vi "CRYSave All.vi"   [LabVIEW 2013]
uses:
  Global/CRYCurve Library Global.vi
panel:
  # "Save All Data(Curves, Values,Results, Waveforms)"
types:
  T1 = cluster{"pattern label":string, "pattern":string}
  T2 = cluster{"pattern label":string, "pattern":string}[]
  T3 = enum16{"Left Button", "Center Button", "Right Button", "Window Close"}
  T4 = typedef "CRYData Cluster.ctl" = cluster{"Name":string, "Curve":cluster{"x":dbl, "y":dbl, "z":dbl}[], "X data":u16, "Y data":u16, "Z data":u16, "X axis":u16, "Y axis":u16, "Z axis":u16, "X unit":string, "Y unit":string, "Z unit":string, "X dB ref":dbl, "Y dB ref":dbl, "Z dB ref":dbl, "single val":bool, "protected":bool, "display X":bool, "display Y":bool, "display Z":bool, "Test Info":string, "Step No.":i32, "Plot Settings":cluster{"Color":u32, "Interpolation":u8, "Point Style":u8, "Line Style":u8, "Point Color":u32, "Line Width":u8, "Bar Plot Style":u8, "Fill To":i16}, "AutoProtect":bool}
  T5 = typedef "CRYWaveform Cluster.ctl" = cluster{"Waveform":cluster{"X0":dbl, "dX":dbl, "Y":sgl[]}, "X data":u16, "Y data":u16, "Y axis":u16, "X unit":string, "Y unit":string, "Y dB ref":dbl, "display Y":bool, "display X":bool, "Overload?":bool, "Test Info":string, "Step No.":i32, "Name":string, "protected":bool, "Sqc history":string[], "Signal Channel ID":i32, "Plot Settings":cluster{"Color":u32, "Interpolation":u8, "Point Style":u8, "Line Style":u8, "Point Color":u32, "Line Width":u8, "Bar Plot Style":u8, "Fill To":i16}, "AutoProtect":bool}
  T6 = typedef "CRYResult Cluster.ctl" = cluster{"Name":string, "Margin":dbl, "unit":string, "Verdict":bool, "Limit":string, "Max/Min":string, "protected":bool, "Step No.":i32, "Test Info":string, "AutoProtect":bool}
  T7 = cluster{"layout":enum16{"rows", "columns"}, "notation":enum16{"sci", "float"}, "precision":i32, "header":enum16{"none", "standard", "custom"}, "custom header":string, "serial no.":bool, "delimiter":enum16{"tab", "comma", "space", "other"}, "other delim":string, "axes":cluster{"x":bool, "y":bool, "z":bool}, "Lot No.":bool, "Operator":bool, "Time Stamp":bool}
  T8 = enum16{"OK", "Yes", "YesNo", "YesNoCancel", "ReplaceAppend"}
  T9 = cluster{"Header format":u16, "Custom Header":string, "Layout":u16, "Delimiter":i32, "Character":string, "notation":u16, "Decimal places":i32, "Comment":string, "axes":cluster{"x":bool, "y":bool, "z":bool}}
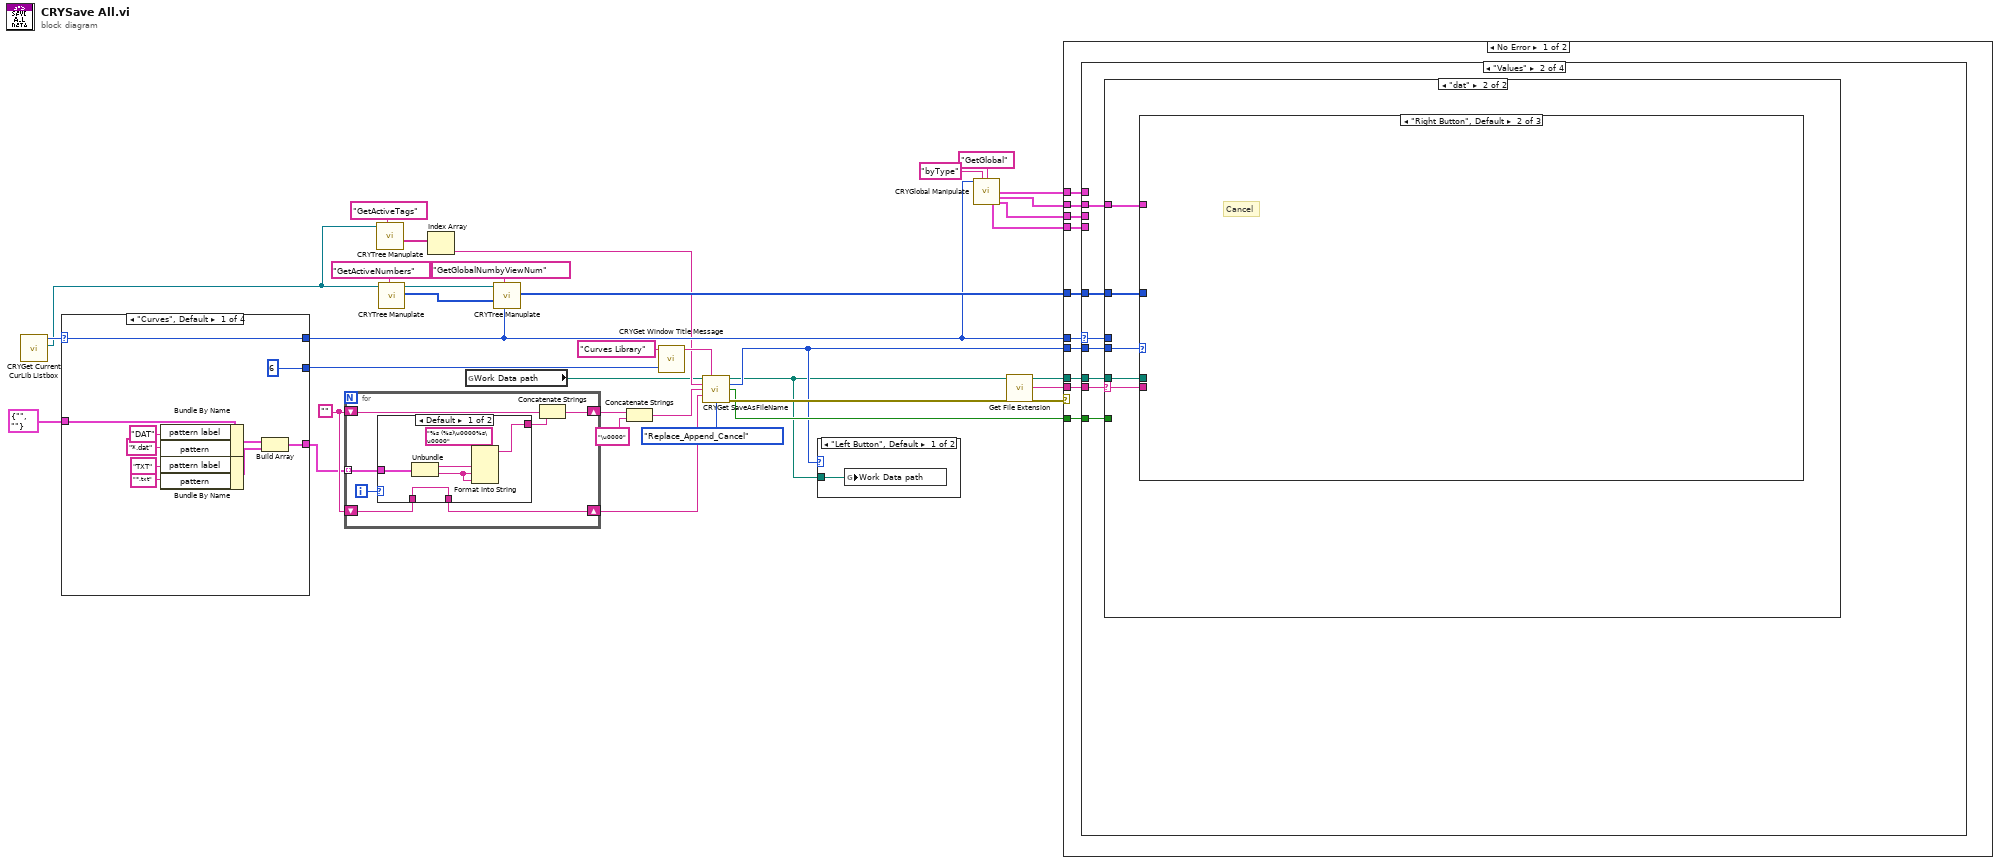
[diagram p0: block diagram]
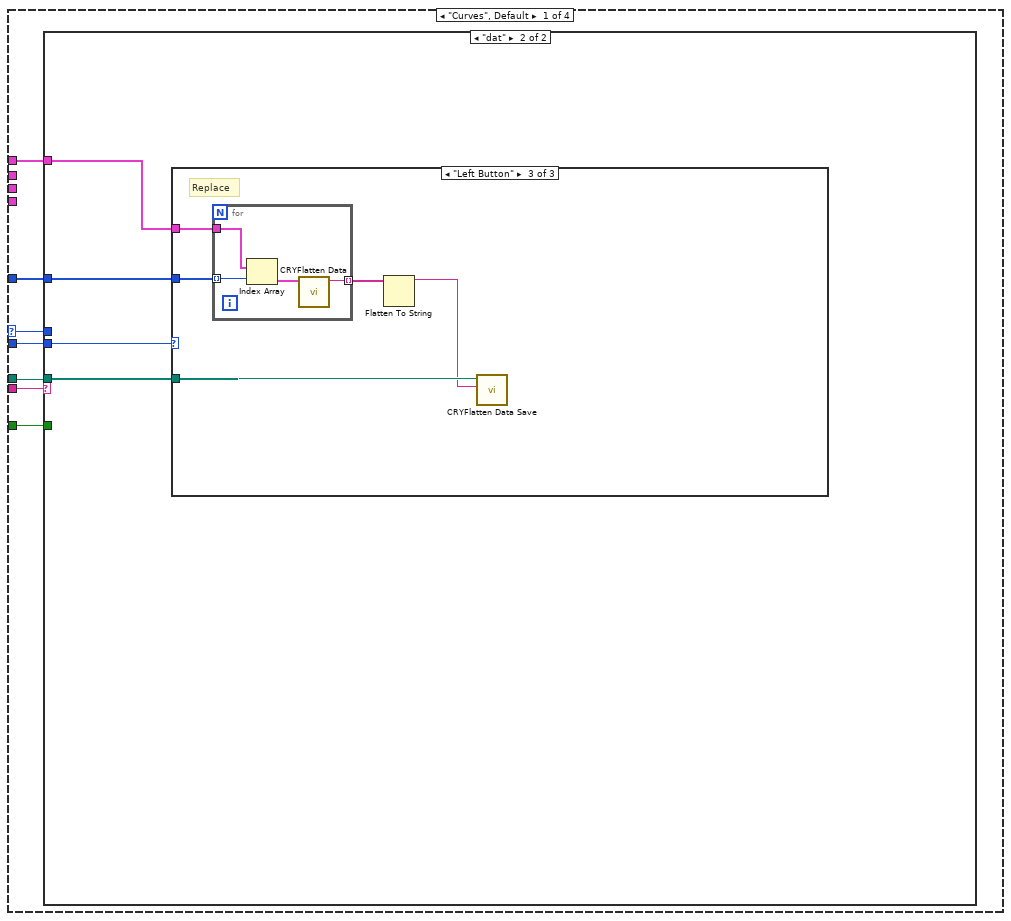
[diagram p3: hidden frame]
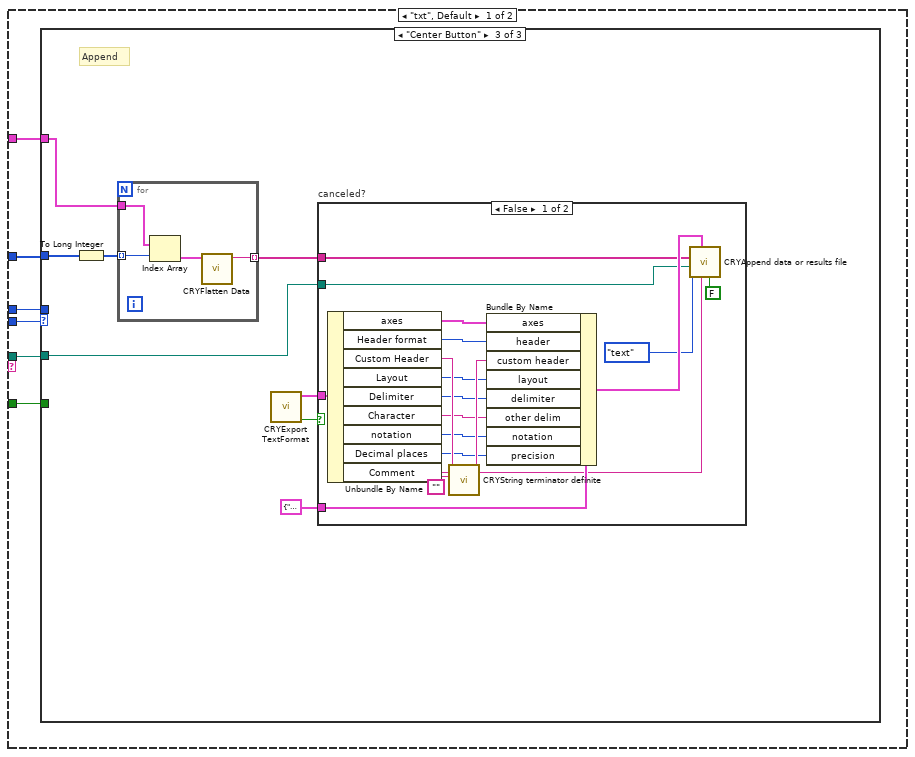
[diagram p4: hidden frame]
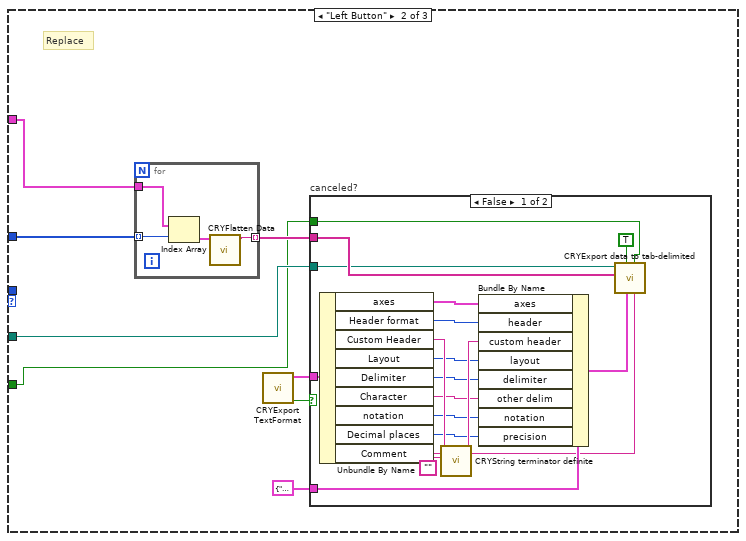
[diagram p6: hidden frame]
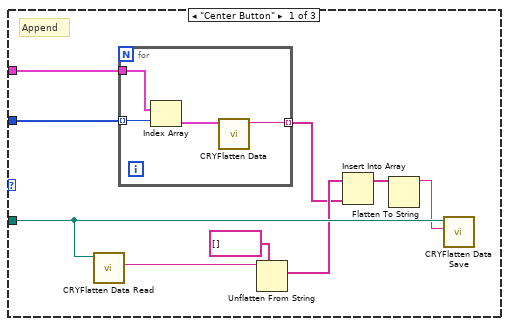
[diagram p9: hidden frame]
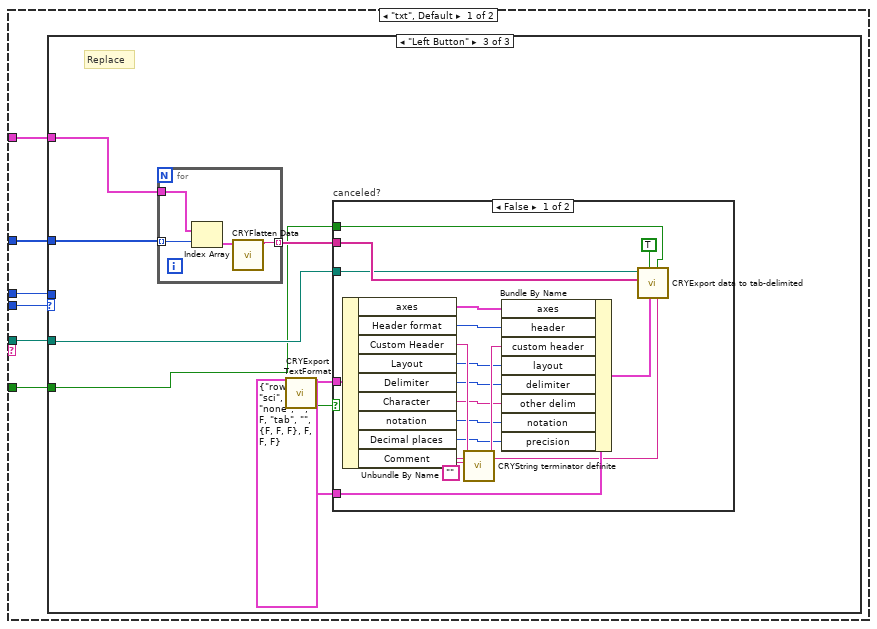
[diagram p11: hidden frame]
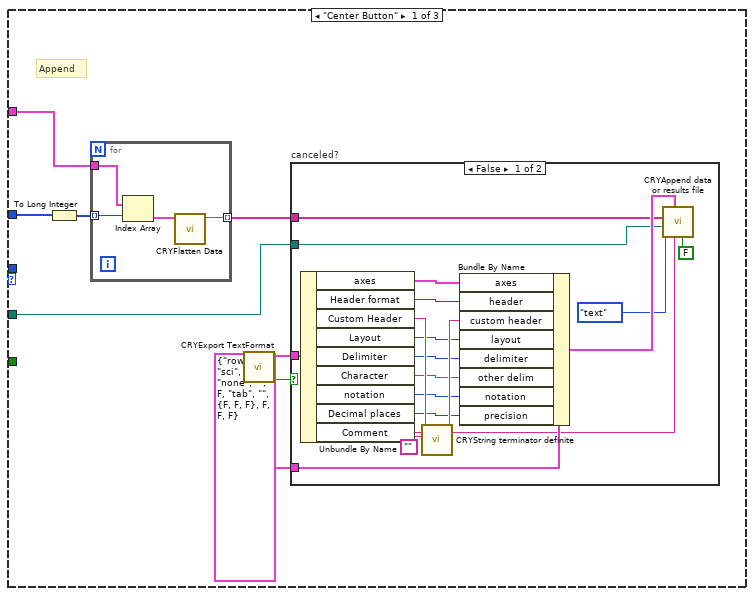
[diagram p12: hidden frame]
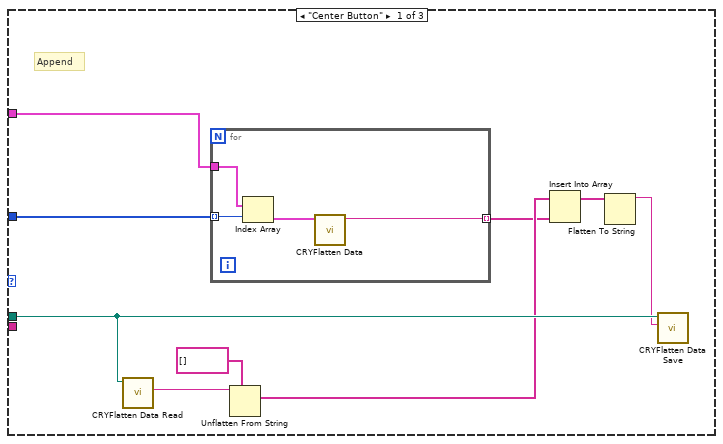
[diagram p16: hidden frame]
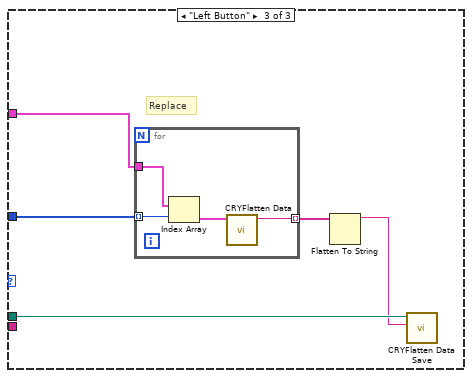
[diagram p17: hidden frame]
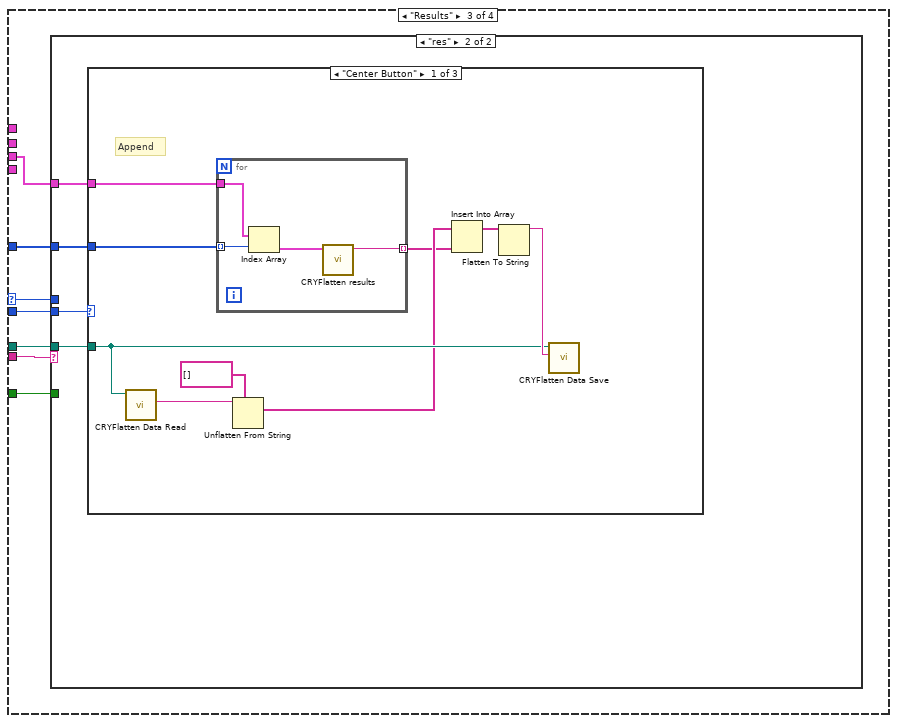
[diagram p18: hidden frame]
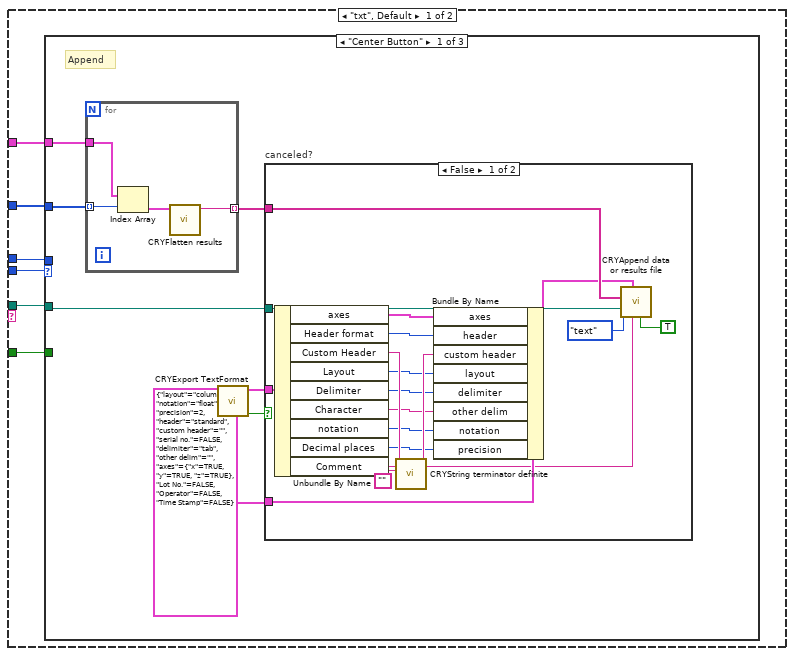
[diagram p19: hidden frame]
diagram:
  w26 = ""
  n1 = call "CRYGet Current CurLib Listbox.vi"() -> ("CurLib Tree"=w6:refnum<vi>, "Type"=w32:enum16{"Curves", "Values", "Results", "WFM"})  [unwired: 9 in, 1 out]
  n2 = case shown="\"Curves\", Default" w32 {
    selector: w32 -> [w46 w56 w66 w76]
    tunnel: [w46 w56 w66 w76] -> w8
    tunnel: [6 ("Error No") 7 ("Error No") 8 ("Error No") 9 ("Error No")] -> w29
    tunnel: T1 {"pattern label"="", "pattern"=""} ("File Types") -> [w37 w47 w58 w68]
    tunnel: [w38 w48 w57 w67] -> w22
    frame "Curves", Default {
      n3 = Bundle By Name(cluster=w37, "pattern label"="DAT" ("pattern (all files)"), "pattern"="*.dat" ("pattern (all files)")) -> (w41:T1)
      n4 = Bundle By Name(cluster=w37, "pattern label"="TXT" ("pattern (all files)"), "pattern"="*.txt" ("pattern (all files)")) -> (w42:T1)
      n5 = Build Array(w41, w42) -> (w38:T2)
    }
    frame "Values" {
      n6 = Bundle By Name(cluster=w47, "pattern label"="DAT" ("pattern (all files)"), "pattern"="*.dat" ("pattern (all files)")) -> (w51:T1)
      n7 = Bundle By Name(cluster=w47, "pattern label"="TXT" ("pattern (all files)"), "pattern"="*.txt" ("pattern (all files)")) -> (w52:T1)
      n8 = Build Array(w51, w52) -> (w48:T2)
    }
    frame "Results" {
      n9 = Bundle By Name(cluster=w58, "pattern label"="RES" ("pattern (all files)"), "pattern"="*.res" ("pattern (all files)")) -> (w61:T1)
      n10 = Bundle By Name(cluster=w58, "pattern label"="TXT" ("pattern (all files)"), "pattern"="*.txt" ("pattern (all files)")) -> (w62:T1)
      n11 = Build Array(w61, w62) -> (w57:T2)
    }
    frame "WFM" {
      n12 = Bundle By Name(cluster=w68, "pattern label"="WAV" ("pattern (all files)"), "pattern"="*.wav" ("pattern (all files)")) -> (w71:T1)
      n13 = Bundle By Name(cluster=w68, "pattern label"="WFM" ("pattern (all files)"), "pattern"="*.wfm" ("pattern (all files)")) -> (w72:T1)
      n14 = Build Array(w71, w72) -> (w67:T2)
    }
  }
  n15 = for {
    tunnel: w22 -> [w83] mode=indexing
    shift-right: [w82] -> w28
    shift-left: w26 -> [w81]
    shift-right: [w78] -> w24
    shift-left: w26 -> [w77]
    i -> [w80]
    n16 = case shown="Default" w80 {
      tunnel: w83 -> [w89 w94]
      tunnel: [w85 w91] -> w79
      tunnel: [w84 w90] -> w78
      tunnel: w77 -> [w84 _]
      frame Default {
        n17 = Unbundle(w89) -> ("pattern label"=w88:string, "pattern"=w86:string)
        n18 = Format Into String(format string="%s (%s)\u0000%s\u0000", w88, w86, w86) -> (resulting string=w85:string)  [unwired: 2 in, 1 out]
      }
      frame 0 {
        n19 = Unbundle(w94) -> ("pattern label"=w90:string, "pattern"=w92:string)
        n20 = Format Into String(format string="%s)\u0000%s\u0000", w92, w92) -> (resulting string=w91:string)  [unwired: 2 in, 1 out]
      }
    }
    n21 = Concatenate Strings(w81, w79) -> (w82:string)
  }
  n22 = call "CRYTree Manuplate.vi"("sAction"="GetActiveTags", "Tree in"=w6) -> ("sData Out"=w5:string[])  [unwired: 6 in, 3 out]
  n23 = call "CRYTree Manuplate.vi"("sAction"="GetActiveNumbers", "Tree in"=w6) -> ("nData Out"=w10:i32[], "Tree Out"=w12:refnum<vi>)  [unwired: 6 in, 2 out]
  n24 = Index Array(array=w5) -> (element=w4:string)  [unwired: 1 in]
  n25 = global read "CRYCurve Library Global.vi" "Work Data path"() -> (w3:path)
  n26 = call "CRYTree Manuplate.vi"("Type"=w8, "sAction"="GetGlobalNumbyViewNum", "nData"=w10, "Tree in"=w12) -> ("nData Out"=w9:i32[])  [unwired: 4 in, 3 out]
  n27 = Concatenate Strings(w28, "\u0000" ("format string")) -> (w25:string)
  n28 = call "CRYGet Window Title Message.vi"("No"=w29, "Kind"="Curves Library") -> ("Multibyte String"=w30:string)  [unwired: 4 in, 5 out]
  n29 = call "CRYGet SaveAsFileName.vi"("Start path"=w3, "TitleName"=w30, "default name"=w4, "pattern (all files)"=w25, "pattern label"=w24, "Enum"=enum16{"Yes_No_Cancel", "Replace_Append_Cancel"}."Replace_Append_Cancel") -> ("Path"=w1:path, "Which Button?"=w2:T3, "Is Replace?"=w21:bool, "error out"=w35:errorcluster)  [unwired: 3 in, 3 out]
  n30 = case shown="\"Left Button\", Default" w2 {
    tunnel: w1 -> [w95 _]
    frame "Left Button", Default {
      n31 = global write "CRYCurve Library Global.vi" "Work Data path"(w95) -> ()
    }
    frame "Right Button" {
    }
  }
  n32 = call "CRYGlobal Manipulate.vi"("Type"=w8, "sOption"="byType", "sAction"="GetGlobal") -> ("Curves Out"=w16:T4[], "Values Out"=w15:T4[], "WFM Out"=w13:T5[], "Results Out"=w14:T6[])  [unwired: 6 in, 3 out]
  n33 = call <vilib>:"Get File Extension.vi"("error in (no error)"=w35, "file"=w1) -> ("error out"=w20:errorcluster, "lowercase file extension"=w33:string, "dup file"=w34:path)  [unwired: 7 out]
  n34 = case shown="No Error" w20 {
    tunnel: w2 -> [w105 _]
    tunnel: w8 -> [w104 _]
    tunnel: w34 -> [w103 _]
    tunnel: w33 -> [w102 _]
    tunnel: w9 -> [w101 _]
    tunnel: w21 -> [w100 _]
    tunnel: w16 -> [w99 _]
    tunnel: w15 -> [w98 _]
    tunnel: w14 -> [w97 _]
    tunnel: w13 -> [w96 _]
    frame No Error {
      n35 = case shown="\"Values\"" w104 {
        selector: w104 -> [w108 w207 w307 _]
        tunnel: w105 -> [w112 w211 w310 w406]
        tunnel: w101 -> [w111 w210 w311 w407]
        tunnel: w103 -> [w110 w209 w309 w405]
        tunnel: w102 -> [w109 w208 w308 w404]
        tunnel: w100 -> [w107 w206 w306 _]
        tunnel: w99 -> [w106 _ _ _]
        tunnel: w98 -> [_ w205 _ _]
        tunnel: w97 -> [_ _ w305 _]
        tunnel: w96 -> [_ _ _ w403]
        frame "Curves", Default {
          n36 = case shown="\"dat\"" w109 {
            tunnel: w112 -> [w117 w182]
            tunnel: w111 -> [w118 w181]
            tunnel: w110 -> [w116 w180]
            tunnel: w108 -> [w115 _]
            tunnel: w107 -> [w114 _]
            tunnel: w106 -> [w113 w179]
            frame "txt", Default {
              n37 = case shown="\"Center Button\"" w117 {
                tunnel: w118 -> [_ w126 w155]
                tunnel: w116 -> [_ w123 w150]
                tunnel: w115 -> [_ _ _]
                tunnel: w114 -> [_ w120 _]
                tunnel: w113 -> [_ w119 w149]
                frame "Right Button", Default {
                  # "Cancel"
                }
                frame "Left Button" {
                  # "Replace"
                  n38 = for {
                    tunnel: w126 -> [w148] mode=indexing
                    tunnel: w119 -> [w147]
                    tunnel: [w145] -> w121 mode=indexing
                    n39 = Index Array(array=w147, index=w148) -> (element=w146:T4)
                    n40 = call "CRYFlatten Data.vi"("Datum"=w146) -> ("Data flattened"=w145:string)  [unwired: 10 in]
                  }
                  n41 = call "CRYExport TextFormat.vi"() -> ("Canceled"=w125:bool, "Export format"=w124:T9)  [unwired: 10 in]
                  n42 = case "canceled?" shown="False" w125 {
                    tunnel: w124 -> [w144 _]
                    tunnel: T7 {"layout"=enum."rows", "notation"=enum."sci", "precision"=0, "header"=enum."none", "custom header"="", "serial no."=FALSE, "delimiter"=enum."tab", "other delim"="", "axes"={"x"=FALSE, "y"=FALSE, "z"=FALSE}, "Lot No."=FALSE, "Operator"=FALSE, "Time Stamp"=FALSE} ("input cluster") -> [w135 _]
                    tunnel: w123 -> [w129 _]
                    tunnel: w121 -> [w130 _]
                    tunnel: w120 -> [w127 _]
                    frame False {
                      n43 = Unbundle By Name(w144) -> ("axes"=w131:cluster{"x":bool, "y":bool, "z":bool}, "Header format"=w136:u16, "Custom Header"=w143:string, "Layout"=w137:u16, "Delimiter"=w138:i32, "Character"=w139:string, "notation"=w140:u16, "Decimal places"=w141:i32, "Comment"=w132:string)
                      n44 = call "CRYString terminator definite.vi"("Terminator"="", "String in"=w143) -> ("String out"=w142:string)  [unwired: 9 in]
                      n45 = Bundle By Name(cluster=w135, "axes"=w131, "header"=w136, "custom header"=w142, "layout"=w137, "delimiter"=w138, "other delim"=w139, "notation"=w140, "precision"=w141) -> (w134:T7)
                      n46 = call "CRYExport data to tab-delimited.vi"("Comment"=w132, "File exists & overwrite (F)"=w127, "Format info"=w134, "Use format info? (F)"=TRUE, "data series"=w130, "File path (not wired: dialogue)"=w129) -> ()  [unwired: 3 in, 3 out]
                    }
                    frame True {
                    }
                  }
                }
                frame "Center Button" {
                  # "Append"
                  n47 = To Long Integer(number=w155) -> (32bit integer=w156:i32[])
                  n48 = for {
                    tunnel: w156 -> [w178] mode=indexing
                    tunnel: w149 -> [w177]
                    tunnel: [w176] -> w151 mode=indexing
                    n49 = Index Array(array=w177, index=w178) -> (element=w175:T4)
                    n50 = call "CRYFlatten Data.vi"("Datum"=w175) -> ("Data flattened"=w176:string)  [unwired: 10 in]
                  }
                  n51 = call "CRYExport TextFormat.vi"() -> ("Canceled"=w154:bool, "Export format"=w153:T9)  [unwired: 10 in]
                  n52 = case "canceled?" shown="False" w154 {
                    tunnel: w153 -> [w174 _]
                    tunnel: T7 {"layout"=enum."rows", "notation"=enum."sci", "precision"=0, "header"=enum."none", "custom header"="", "serial no."=FALSE, "delimiter"=enum."tab", "other delim"="", "axes"={"x"=FALSE, "y"=FALSE, "z"=FALSE}, "Lot No."=FALSE, "Operator"=FALSE, "Time Stamp"=FALSE} ("input cluster") -> [w165 _]
                    tunnel: w150 -> [w157 _]
                    tunnel: w151 -> [w160 _]
                    frame False {
                      n53 = Unbundle By Name(w174) -> ("axes"=w161:cluster{"x":bool, "y":bool, "z":bool}, "Header format"=w166:u16, "Custom Header"=w173:string, "Layout"=w167:u16, "Delimiter"=w168:i32, "Character"=w169:string, "notation"=w170:u16, "Decimal places"=w171:i32, "Comment"=w162:string)
                      n54 = call "CRYString terminator definite.vi"("Terminator"="", "String in"=w173) -> ("String out"=w172:string)  [unwired: 9 in]
                      n55 = Bundle By Name(cluster=w165, "axes"=w161, "header"=w166, "custom header"=w172, "layout"=w167, "delimiter"=w168, "other delim"=w169, "notation"=w170, "precision"=w171) -> (w164:T7)
                      n56 = call "CRYAppend data or results file.vi"("Is results? (F)"=FALSE, "Comment"=w162, "Format info"=w164, "data format"=enum16{"text", "DAT"}."text", "Datafile path"=w157, "Curves list to save"=w160) -> ()  [unwired: 5 in, 1 out]
                    }
                    frame True {
                    }
                  }
                }
              }
            }
            frame "dat" {
              n57 = case shown="\"Left Button\"" w182 {
                tunnel: w181 -> [w191 _ w200]
                tunnel: w179 -> [w185 _ w198]
                tunnel: w180 -> [w190 _ w197]
                frame "Center Button" {
                  # "Append"
                  n58 = call "CRYFlatten Data Read.vi"("Path In"=w190) -> ("Flatten Data Out"=w189:string)  [unwired: 1 in, 7 out]
                  n59 = for {
                    tunnel: w191 -> [w195] mode=indexing
                    tunnel: w185 -> [w194]
                    tunnel: [w192] -> w184 mode=indexing
                    n60 = Index Array(array=w194, index=w195) -> (element=w193:T4)
                    n61 = call "CRYFlatten Data.vi"("Datum"=w193) -> ("Data flattened"=w192:string)  [unwired: 10 in]
                  }
                  n62 = Unflatten From String(type=string[] [] ("value"), binary string=w189) -> (value=w186:string[])  [unwired: 1 in, 4 out]
                  n63 = Insert Into Array(array=w186, new element=w184) -> (w187:string[])  [unwired: 1 in]
                  n64 = Flatten To String(anything=w187) -> (data string=w188:string)  [unwired: 1 in, 4 out]
                  n65 = call "CRYFlatten Data Save.vi"("Any Flatten Data"=w188, "Path In"=w190) -> ()  [unwired: 1 in, 7 out]
                }
                frame "Right Button", Default {
                  # "Cancel"
                }
                frame "Left Button" {
                  # "Replace"
                  n66 = for {
                    tunnel: w200 -> [w204] mode=indexing
                    tunnel: w198 -> [w203]
                    tunnel: [w201] -> w199 mode=indexing
                    n67 = Index Array(array=w203, index=w204) -> (element=w202:T4)
                    n68 = call "CRYFlatten Data.vi"("Datum"=w202) -> ("Data flattened"=w201:string)  [unwired: 10 in]
                  }
                  n69 = Flatten To String(anything=w199) -> (data string=w196:string)  [unwired: 1 in, 4 out]
                  n70 = call "CRYFlatten Data Save.vi"("Any Flatten Data"=w196, "Path In"=w197) -> ()  [unwired: 1 in, 7 out]
                }
              }
            }
          }
        }
        frame "Values" {
          n71 = case shown="\"dat\"" w208 {
            selector: w208 -> [_ w278]
            tunnel: w211 -> [w217 w282]
            tunnel: w210 -> [w214 w281]
            tunnel: w209 -> [w216 w280]
            tunnel: w207 -> [w215 _]
            tunnel: w206 -> [w213 _]
            tunnel: w205 -> [w212 w279]
            frame "txt", Default {
              n72 = case shown="\"Left Button\"" w217 {
                tunnel: w214 -> [w219 _ w251]
                tunnel: w216 -> [w220 _ w250]
                tunnel: w215 -> [_ _ _]
                tunnel: w213 -> [_ _ w249]
                tunnel: w212 -> [w218 _ w248]
                frame "Center Button" {
                  # "Append"
                  n73 = To Long Integer(number=w219) -> (32bit integer=w225:i32[])
                  n74 = for {
                    tunnel: w225 -> [w247] mode=indexing
                    tunnel: w218 -> [w246]
                    tunnel: [w245] -> w221 mode=indexing
                    n75 = Index Array(array=w246, index=w247) -> (element=w244:T4)
                    n76 = call "CRYFlatten Data.vi"("Datum"=w244) -> ("Data flattened"=w245:string)  [unwired: 10 in]
                  }
                  n77 = call "CRYExport TextFormat.vi"() -> ("Canceled"=w224:bool, "Export format"=w223:T9)  [unwired: 10 in]
                  n78 = case "canceled?" shown="False" w224 {
                    tunnel: w223 -> [w243 _]
                    tunnel: T7 {"layout"=enum."rows", "notation"=enum."sci", "precision"=0, "header"=enum."none", "custom header"="", "serial no."=FALSE, "delimiter"=enum."tab", "other delim"="", "axes"={"x"=FALSE, "y"=FALSE, "z"=FALSE}, "Lot No."=FALSE, "Operator"=FALSE, "Time Stamp"=FALSE} ("input cluster") -> [w234 _]
                    tunnel: w220 -> [w226 _]
                    tunnel: w221 -> [w229 _]
                    frame False {
                      n79 = Unbundle By Name(w243) -> ("axes"=w230:cluster{"x":bool, "y":bool, "z":bool}, "Header format"=w235:u16, "Custom Header"=w242:string, "Layout"=w236:u16, "Delimiter"=w237:i32, "Character"=w238:string, "notation"=w239:u16, "Decimal places"=w240:i32, "Comment"=w231:string)
                      n80 = call "CRYString terminator definite.vi"("Terminator"="", "String in"=w242) -> ("String out"=w241:string)  [unwired: 9 in]
                      n81 = Bundle By Name(cluster=w234, "axes"=w230, "header"=w235, "custom header"=w241, "layout"=w236, "delimiter"=w237, "other delim"=w238, "notation"=w239, "precision"=w240) -> (w233:T7)
                      n82 = call "CRYAppend data or results file.vi"("Is results? (F)"=FALSE, "Comment"=w231, "Format info"=w233, "data format"=enum16{"text", "DAT"}."text", "Datafile path"=w226, "Curves list to save"=w229) -> ()  [unwired: 5 in, 1 out]
                    }
                    frame True {
                    }
                  }
                }
                frame "Right Button", Default {
                  # "Cancel"
                }
                frame "Left Button" {
                  # "Replace"
                  n83 = for {
                    tunnel: w251 -> [w277] mode=indexing
                    tunnel: w248 -> [w276]
                    tunnel: [w274] -> w252 mode=indexing
                    n84 = Index Array(array=w276, index=w277) -> (element=w275:T4)
                    n85 = call "CRYFlatten Data.vi"("Datum"=w275) -> ("Data flattened"=w274:string)  [unwired: 10 in]
                  }
                  n86 = call "CRYExport TextFormat.vi"() -> ("Canceled"=w255:bool, "Export format"=w254:T9)  [unwired: 10 in]
                  n87 = case "canceled?" shown="False" w255 {
                    tunnel: w254 -> [w273 _]
                    tunnel: T7 {"layout"=enum."rows", "notation"=enum."sci", "precision"=0, "header"=enum."none", "custom header"="", "serial no."=FALSE, "delimiter"=enum."tab", "other delim"="", "axes"={"x"=FALSE, "y"=FALSE, "z"=FALSE}, "Lot No."=FALSE, "Operator"=FALSE, "Time Stamp"=FALSE} ("input cluster") -> [w264 _]
                    tunnel: w250 -> [w258 _]
                    tunnel: w252 -> [w259 _]
                    tunnel: w249 -> [w256 _]
                    frame False {
                      n88 = Unbundle By Name(w273) -> ("axes"=w260:cluster{"x":bool, "y":bool, "z":bool}, "Header format"=w265:u16, "Custom Header"=w272:string, "Layout"=w266:u16, "Delimiter"=w267:i32, "Character"=w268:string, "notation"=w269:u16, "Decimal places"=w270:i32, "Comment"=w261:string)
                      n89 = call "CRYString terminator definite.vi"("Terminator"="", "String in"=w272) -> ("String out"=w271:string)  [unwired: 9 in]
                      n90 = Bundle By Name(cluster=w264, "axes"=w260, "header"=w265, "custom header"=w271, "layout"=w266, "delimiter"=w267, "other delim"=w268, "notation"=w269, "precision"=w270) -> (w263:T7)
                      n91 = call "CRYExport data to tab-delimited.vi"("Comment"=w261, "File exists & overwrite (F)"=w256, "Format info"=w263, "Use format info? (F)"=TRUE, "data series"=w259, "File path (not wired: dialogue)"=w258) -> ()  [unwired: 3 in, 3 out]
                    }
                    frame True {
                    }
                  }
                }
              }
            }
            frame "dat" {
              n92 = case shown="\"Right Button\", Default" w282 {
                tunnel: w281 -> [w291 _ w300]
                tunnel: w280 -> [w289 _ w298]
                tunnel: w279 -> [w283 _ w296]
                tunnel: w278 -> [_ _ _]
                frame "Center Button" {
                  # "Append"
                  n93 = call "CRYFlatten Data Read.vi"("Path In"=w289) -> ("Flatten Data Out"=w290:string)  [unwired: 1 in, 7 out]
                  n94 = for {
                    tunnel: w291 -> [w295] mode=indexing
                    tunnel: [w292] -> w284 mode=indexing
                    tunnel: w283 -> [w294]
                    n95 = Index Array(array=w294, index=w295) -> (element=w293:T4)
                    n96 = call "CRYFlatten Data.vi"("Datum"=w293) -> ("Data flattened"=w292:string)  [unwired: 10 in]
                  }
                  n97 = Unflatten From String(type=string[] [] ("value"), binary string=w290) -> (value=w285:string[])  [unwired: 1 in, 4 out]
                  n98 = Insert Into Array(array=w285, new element=w284) -> (w287:string[])  [unwired: 1 in]
                  n99 = Flatten To String(anything=w287) -> (data string=w288:string)  [unwired: 1 in, 4 out]
                  n100 = call "CRYFlatten Data Save.vi"("Any Flatten Data"=w288, "Path In"=w289) -> ()  [unwired: 1 in, 7 out]
                }
                frame "Right Button", Default {
                  # "Cancel"
                }
                frame "Left Button" {
                  # "Replace"
                  n101 = for {
                    tunnel: w300 -> [w304] mode=indexing
                    tunnel: [w301] -> w299 mode=indexing
                    tunnel: w296 -> [w303]
                    n102 = Index Array(array=w303, index=w304) -> (element=w302:T4)
                    n103 = call "CRYFlatten Data.vi"("Datum"=w302) -> ("Data flattened"=w301:string)  [unwired: 10 in]
                  }
                  n104 = Flatten To String(anything=w299) -> (data string=w297:string)  [unwired: 1 in, 4 out]
                  n105 = call "CRYFlatten Data Save.vi"("Any Flatten Data"=w297, "Path In"=w298) -> ()  [unwired: 1 in, 7 out]
                }
              }
            }
          }
        }
        frame "Results" {
          n106 = case shown="\"res\"" w308 {
            tunnel: w305 -> [w317 w380]
            tunnel: w311 -> [w316 w379]
            tunnel: w310 -> [w315 w378]
            tunnel: w309 -> [w313 w377]
            tunnel: w307 -> [w314 _]
            tunnel: w306 -> [w312 _]
            frame "txt", Default {
              n107 = case shown="\"Center Button\"" w315 {
                tunnel: w316 -> [w324 _ w354]
                tunnel: w317 -> [w323 _ w353]
                tunnel: w313 -> [w319 _ w350]
                tunnel: w314 -> [_ _ _]
                tunnel: w312 -> [_ _ w347]
                frame "Center Button" {
                  # "Append"
                  n108 = for {
                    tunnel: w324 -> [w346] mode=indexing
                    tunnel: w323 -> [w345]
                    tunnel: [w343] -> w320 mode=indexing
                    n109 = Index Array(array=w345, index=w346) -> (element=w344:T6)
                    n110 = call "CRYFlatten results.vi"("Result in"=w344) -> ("Flatten Result"=w343:string)  [unwired: 10 in]
                  }
                  n111 = call "CRYExport TextFormat.vi"() -> ("Canceled"=w322:bool, "Export format"=w321:T9)  [unwired: 10 in]
                  n112 = case "canceled?" shown="False" w322 {
                    tunnel: w321 -> [w342 _]
                    tunnel: T7 {"layout"=enum."columns", "notation"=enum."float", "precision"=2, "header"=enum."standard", "custom header"="", "serial no."=FALSE, "delimiter"=enum."tab", "other delim"="", "axes"={"x"=TRUE, "y"=TRUE, "z"=TRUE}, "Lot No."=FALSE, "Operator"=FALSE, "Time Stamp"=FALSE} ("Format info") -> [w333 _]
                    tunnel: w319 -> [w326 _]
                    tunnel: w320 -> [w329 _]
                    frame False {
                      n113 = Unbundle By Name(w342) -> ("axes"=w330:cluster{"x":bool, "y":bool, "z":bool}, "Header format"=w334:u16, "Custom Header"=w341:string, "Layout"=w335:u16, "Delimiter"=w336:i32, "Character"=w337:string, "notation"=w338:u16, "Decimal places"=w339:i32, "Comment"=w331:string)
                      n114 = call "CRYString terminator definite.vi"("Terminator"="", "String in"=w341) -> ("String out"=w340:string)  [unwired: 9 in]
                      n115 = Bundle By Name(cluster=w333, "axes"=w330, "header"=w334, "custom header"=w340, "layout"=w335, "delimiter"=w336, "other delim"=w337, "notation"=w338, "precision"=w339) -> (w325:T7)
                      n116 = call "CRYAppend data or results file.vi"("Is results? (F)"=TRUE, "Comment"=w331, "Format info"=w325, "data format"=enum16{"text", "DAT"}."text", "Datafile path"=w326, "Curves list to save"=w329) -> ()  [unwired: 5 in, 1 out]
                    }
                    frame True {
                    }
                  }
                }
                frame "Right Button", Default {
                  # "Cancel"
                }
                frame "Left Button" {
                  # "Replace"
                  n117 = for {
                    tunnel: w354 -> [w376] mode=indexing
                    tunnel: w353 -> [w375]
                    tunnel: [w373] -> w349 mode=indexing
                    n118 = Index Array(array=w375, index=w376) -> (element=w374:T6)
                    n119 = call "CRYFlatten results.vi"("Result in"=w374) -> ("Flatten Result"=w373:string)  [unwired: 10 in]
                  }
                  n120 = call "CRYExport TextFormat.vi"() -> ("Canceled"=w352:bool, "Export format"=w351:T9)  [unwired: 10 in]
                  n121 = case "canceled?" shown="False" w352 {
                    tunnel: w351 -> [w372 _]
                    tunnel: T7 {"layout"=enum."rows", "notation"=enum."sci", "precision"=0, "header"=enum."none", "custom header"="", "serial no."=FALSE, "delimiter"=enum."tab", "other delim"="", "axes"={"x"=FALSE, "y"=FALSE, "z"=FALSE}, "Lot No."=FALSE, "Operator"=FALSE, "Time Stamp"=FALSE} ("Format info") -> [w363 _]
                    tunnel: w350 -> [w356 _]
                    tunnel: w349 -> [w358 _]
                    tunnel: w347 -> [w355 _]
                    frame False {
                      n122 = Unbundle By Name(w372) -> ("axes"=w360:cluster{"x":bool, "y":bool, "z":bool}, "Header format"=w364:u16, "Custom Header"=w371:string, "Layout"=w365:u16, "Delimiter"=w366:i32, "Character"=w367:string, "notation"=w368:u16, "Decimal places"=w369:i32, "Comment"=w361:string)
                      n123 = call "CRYString terminator definite.vi"("Terminator"="", "String in"=w371) -> ("String out"=w370:string)  [unwired: 9 in]
                      n124 = Bundle By Name(cluster=w363, "axes"=w360, "header"=w364, "custom header"=w370, "layout"=w365, "delimiter"=w366, "other delim"=w367, "notation"=w368, "precision"=w369) -> (w357:T7)
                      n125 = call "CRYResult save as text.vi"("File exists & overwrite (F)"=w355, "Comment"=w361, "File format"=enum16{"text", "RES"}."text", "Format info"=w357, "Path"=w356, "Results stack, flat"=w358) -> ()  [unwired: 6 in]
                    }
                    frame True {
                    }
                  }
                }
              }
            }
            frame "res" {
              n126 = case shown="\"Center Button\"" w378 {
                tunnel: w379 -> [w389 _ w398]
                tunnel: w380 -> [w385 _ w396]
                tunnel: w377 -> [w386 _ w395]
                frame "Center Button" {
                  # "Append"
                  n127 = call "CRYFlatten Data Read.vi"("Path In"=w386) -> ("Flatten Data Out"=w387:string)  [unwired: 1 in, 7 out]
                  n128 = for {
                    tunnel: w389 -> [w393] mode=indexing
                    tunnel: [w391] -> w382 mode=indexing
                    tunnel: w385 -> [w392]
                    n129 = Index Array(array=w392, index=w393) -> (element=w390:T6)
                    n130 = call "CRYFlatten results.vi"("Result in"=w390) -> ("Flatten Result"=w391:string)  [unwired: 10 in]
                  }
                  n131 = Unflatten From String(type=string[] [] ("value"), binary string=w387) -> (value=w383:string[])  [unwired: 1 in, 4 out]
                  n132 = Insert Into Array(array=w383, new element=w382) -> (w384:string[])  [unwired: 1 in]
                  n133 = Flatten To String(anything=w384) -> (data string=w388:string)  [unwired: 1 in, 4 out]
                  n134 = call "CRYFlatten Data Save.vi"("Any Flatten Data"=w388, "Path In"=w386) -> ()  [unwired: 1 in, 7 out]
                }
                frame "Right Button", Default {
                  # "Cancel"
                }
                frame "Left Button" {
                  # "Replace"
                  n135 = for {
                    tunnel: w398 -> [w402] mode=indexing
                    tunnel: [w399] -> w397 mode=indexing
                    tunnel: w396 -> [w401]
                    n136 = Index Array(array=w401, index=w402) -> (element=w400:T6)
                    n137 = call "CRYFlatten results.vi"("Result in"=w400) -> ("Flatten Result"=w399:string)  [unwired: 10 in]
                  }
                  n138 = Flatten To String(anything=w397) -> (data string=w394:string)  [unwired: 1 in, 4 out]
                  n139 = call "CRYFlatten Data Save.vi"("Any Flatten Data"=w394, "Path In"=w395) -> ()  [unwired: 1 in, 7 out]
                }
              }
            }
          }
        }
        frame "WFM" {
          n140 = case shown="\"wav\", Default" w404 {
            tunnel: w403 -> [w411 w460]
            tunnel: w407 -> [w410 w459]
            tunnel: w406 -> [w409 w458]
            tunnel: w405 -> [w408 w457]
            frame "wav", Default {
              n141 = case shown="\"Left Button\"" w409 {
                tunnel: w410 -> [_ _ w418]
                tunnel: w411 -> [_ _ w420]
                tunnel: w408 -> [_ _ w419]
                frame "Center Button" {
                  n142 = call "CRYGet Error Message.vi"("Error No"=5, "Kind"="Curves Library") -> ("Message"=w412:string, "Window Title"=w413:string)  [unwired: 4 in, 4 out]
                  n143 = call "CRYMessage Dialog.vi"("Window Title"=w413, "YesNoCancel"=T8."OK", "Message Content"=w412) -> ()  [unwired: 7 in, 2 out]
                }
                frame "Right Button", Default {
                  # "Cancel"
                }
                frame "Left Button" {
                  # "Replace"
                  n144 = Array Size(array=w418) -> (size(s)=w417:i32)
                  n145 = case shown="1, 2" w417 {
                    selector: w417 -> [w425 _]
                    tunnel: w418 -> [w421 _]
                    tunnel: w420 -> [w426 _]
                    tunnel: w419 -> [w428 _]
                    frame 1, 2 {
                      n146 = case shown="1, Default" w425 {
                        tunnel: [w437 w450] -> w429
                        tunnel: w426 -> [w436 w449]
                        tunnel: [w435 w446] -> w424
                        tunnel: [u32 1 ("Channel") u32 2 ("Channel")] -> w422
                        tunnel: w421 -> [w433 w444]
                        frame 1, Default {
                          n147 = Index Array(array=w433) -> (element=w432:i32)  [unwired: 1 in]
                          n148 = Index Array(array=w436, index=w432) -> (element=w438:T5)
                          n149 = Unbundle By Name(w438) -> ("Waveform.dX"=w437:dbl, "Waveform.Y"=w435:sgl[])
                        }
                        frame 2 {
                          n150 = Index Array(array=w444, index #1=0 ("index"), index #2=1 ("index")) -> (element #1=w443:i32, element #2=w441:i32)
                          n151 = Index Array(array=w449, index #1=w443, index #2=w441) -> (element #1=w451:T5, element #2=w442:T5)
                          n152 = Unbundle By Name(w451) -> ("Waveform.dX"=w450:dbl, "Waveform.Y"=w448:sgl[])
                          n153 = Unbundle By Name(w442) -> ("Waveform.Y"=w447:sgl[])
                          n154 = Interleave 1D Arrays(w448, w447) -> (w446:sgl[])
                        }
                      }
                      n155 = Reciprocal(x=w429) -> (1/x=w427:dbl)
                      n156 = call "CRYSave Wave File.vi"("Channel"=w422, "Wave Data In"=w424, "Sampling Freq"=w427, "Wave File Path In"=w428) -> ("Error Out(0-OK)"=w423:u32)  [unwired: 7 in]
                      n157 = case shown="Default" w423 {
                        frame Default {
                          n158 = call "CRYGet Error Message.vi"("Error No"=4, "Kind"="Curves Library") -> ()  [unwired: 4 in, 6 out]
                        }
                        frame 0 {
                        }
                      }
                    }
                    frame 3.., Default {
                      n159 = call "CRYGet Error Message.vi"("Error No"=3, "Kind"="Curves Library") -> ("Message"=w452:string, "Window Title"=w453:string)  [unwired: 4 in, 4 out]
                      n160 = call "CRYMessage Dialog.vi"("Window Title"=w453, "YesNoCancel"=T8."OK", "Message Content"=w452) -> ()  [unwired: 7 in, 2 out]
                    }
                  }
                }
              }
            }
            frame "wfm" {
              n161 = case shown="\"Center Button\"" w458 {
                tunnel: w459 -> [w469 _ w478]
                tunnel: w460 -> [w467 _ w476]
                tunnel: w457 -> [w466 _ w475]
                frame "Center Button" {
                  # "Append"
                  n162 = call "CRYFlatten Data Read.vi"("Path In"=w466) -> ("Flatten Data Out"=w465:string)  [unwired: 1 in, 7 out]
                  n163 = for {
                    tunnel: w469 -> [w473] mode=indexing
                    tunnel: [w470] -> w461 mode=indexing
                    tunnel: w467 -> [w472]
                    n164 = Index Array(array=w472, index=w473) -> (element=w471:T5)
                    n165 = call "CRYFlatten waveform.vi"("Waveform Cluster"=w471) -> ("Flatten Waveform"=w470:string)  [unwired: 10 in]
                  }
                  n166 = Unflatten From String(type=string[] [] ("value"), binary string=w465) -> (value=w462:string[])  [unwired: 1 in, 4 out]
                  n167 = Insert Into Array(array=w462, new element=w461) -> (w464:string[])  [unwired: 1 in]
                  n168 = Flatten To String(anything=w464) -> (data string=w468:string)  [unwired: 1 in, 4 out]
                  n169 = call "CRYFlatten Data Save.vi"("Any Flatten Data"=w468, "Path In"=w466) -> ()  [unwired: 1 in, 7 out]
                }
                frame "Right Button", Default {
                  # "Cancel"
                }
                frame "Left Button" {
                  # "Replace"
                  n170 = for {
                    tunnel: w478 -> [w482] mode=indexing
                    tunnel: [w479] -> w477 mode=indexing
                    tunnel: w476 -> [w481]
                    n171 = Index Array(array=w481, index=w482) -> (element=w480:T5)
                    n172 = call "CRYFlatten waveform.vi"("Waveform Cluster"=w480) -> ("Flatten Waveform"=w479:string)  [unwired: 10 in]
                  }
                  n173 = Flatten To String(anything=w477) -> (data string=w474:string)  [unwired: 1 in, 4 out]
                  n174 = call "CRYFlatten Data Save.vi"("Any Flatten Data"=w474, "Path In"=w475) -> ()  [unwired: 1 in, 7 out]
                }
              }
            }
          }
        }
      }
    }
    frame Error {
    }
  }
